vi "correct file path.vi"(8 "error in (no error)":errorcluster, 10 "replacement (-)":string="-", 11 "input path":string) -> (0 "error out":errorcluster, 3 "corrected path":string)   [LabVIEW 2017]
doc: "Replaces invalid characters in file path with valid a character.\nreplacement - default is \"space\""
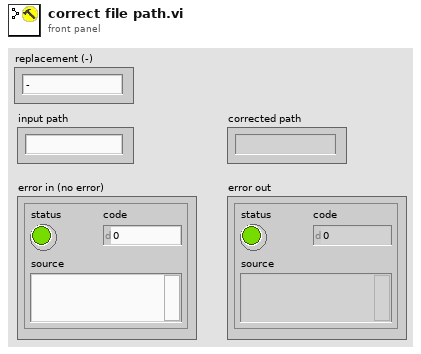
[diagram p1: front panel]
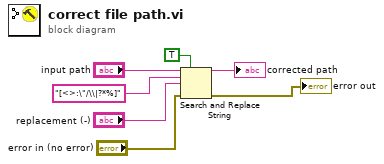
[diagram p0: block diagram]
diagram:
  n1 = Search and Replace String(replace all?=TRUE ("replace all? (F)"), input string="input path", search string="[<>:\"/\\|?*%]" ("regular expression"), replace string="replacement (-)", error in="error in (no error)") -> (result string=→"corrected path":string, error out=→"error out":errorcluster)  [unwired: 3 in, 2 out]
